vi "Remove.vi"(8 "error in (no error)":errorcluster, 10 "Key":variant, 11 "Store in":refnum<class "Store.lvclass">) -> (0 "error out":errorcluster, 1 "Success?":bool, 3 "Store out":refnum<class "Store.lvclass">)   [LabVIEW 2018, in "Application.lvlib" / "Store.lvclass"]
uses:
  Store.lvclass
  Store.lvclass/Store.ctl
  Dictionary Class/Dictionary.lvclass/Dictionary.ctl
  Dictionary Class/VIs/Get Data DVR.vi
  Dictionary Class/Dictionary.lvclass
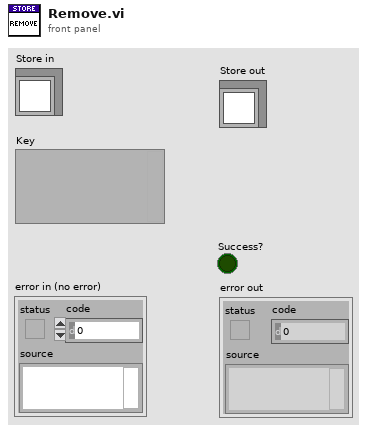
[diagram p1: front panel]
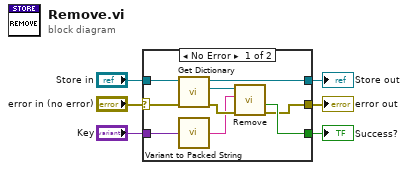
[diagram p0: block diagram]
diagram:
  n1 = case shown="No Error" "error in (no error)" {
    selector: "error in (no error)" -> [w14 w17]
    tunnel: [w7 w17] -> w5
    tunnel: [w12 w16] -> w3
    tunnel: "Store in" -> [w15 w16]
    tunnel: "Key" -> [w13 _]
    tunnel: [w8 _] -> w1
    frame No Error {
      n2 = call "Get Dictionary.vi"("error in (no error)"=w14, "Store in"=w15) -> ("error out"=w10:errorcluster, "Dictionary.lvclass"=w11:refnum<class "Dictionary.lvclass">, "Store out"=w12:refnum<class "Store.lvclass">)  [unwired: 7 in]
      n3 = call "Variant to Packed String.vi"("Variant"=w13) -> ("Packed String"=w9:string)  [unwired: 3 in, 1 out]
      n4 = call "Remove.vi"("error in (no error)"=w10, "Key"=w9, "Dictionary in"=w11) -> ("error out"=w7:errorcluster, "Success?"=w8:bool)  [unwired: 6 in, 1 out]
    }
    frame Error {
    }
  }
  "error out" <- w5
  "Store out" <- w3
  "Success?" <- w1
